vi "Error output.vi"(7 "Actions":T1=enum."Clear", 10 "time":dbl format="%#_13g", 11 "Error In":errorcluster) -> (1 "max time":dbl, 2 "average time":dbl, 3 "Error Out":errorcluster)   [LabVIEW 2018]
uses:
  Controls/FGV Actions.ctl
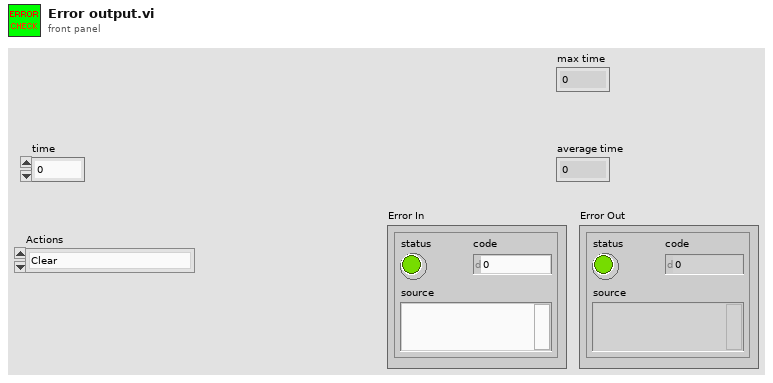
[diagram p1: front panel]
types:
  T1 = typedef "FGV Actions.ctl" = enum16{"Init", "Set", "Get", "Clear"}
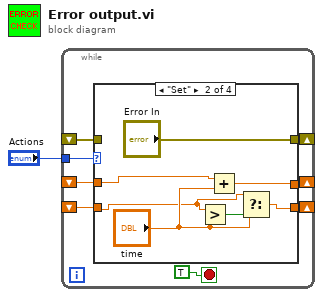
[diagram p0: block diagram]
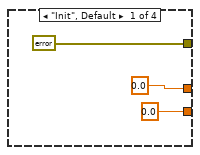
[diagram p2: hidden frame]
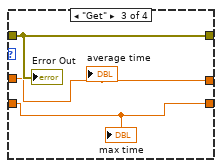
[diagram p3: hidden frame]
diagram:
  n1 = while {
    tunnel: "Actions" -> [w8]
    shift-right: [w7] -> _
    shift-left: _ -> [w6]
    shift-right: [w5] -> _
    shift-left: _ -> [w4]
    shift-right: [w3] -> _
    shift-left: _ -> [w2]
    stop <- TRUE stop-if-true
    n2 = case shown="\"Set\"" w8 {
      tunnel: [errorcluster {"status"=FALSE, "code"=0, "source"=""} ("error constant") "Error In" w22 _] -> w7
      tunnel: w6 -> [_ _ w22 _]
      tunnel: [0.0 ("time") w18 w21 _] -> w5
      tunnel: w4 -> [_ w16 w21 _]
      tunnel: [0.0 ("time") w14 w20 _] -> w3
      tunnel: w2 -> [_ w13 w20 _]
      frame "Init", Default {
      }
      frame "Set" {
        n3 = Greater?(x=w13, y="time") -> (0:w17:bool)
        n4 = Add(x=w16, y="time") -> (x+y=w18:dbl)
        n5 = Select(t=w13, s=w17, f="time") -> (s? t:f=w14:dbl)
      }
      frame "Get" {
        "Error Out" <- w22
        "average time" <- w21
        "max time" <- w20
      }
      frame "Clear" {
      }
    }
  }
